vi "sort and index.vi"(2 "Reverse":bool, 3 "Array to Sort":string[](array[string])) -> (0 "Sorted Indices Array":i32[](array[numeric]), 1 "Sorted Array":string[](array[string]))   [LabVIEW 2015]
doc: "This example VI will sort a 1D array and provide an Index Matrix.\n\nFor example:\n\nunsorted array A=[5 4 5 3 1 2]\nsorted array B = [1 2 3 4 5 5]\nIndex Array = [4 5 3 1 0 2]"
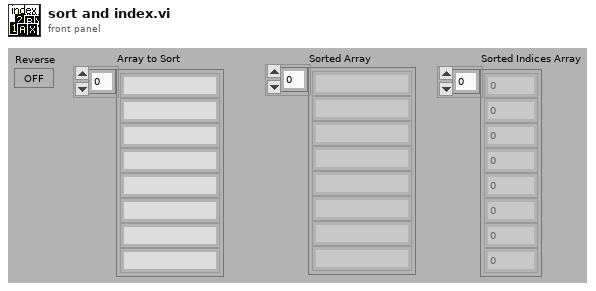
[diagram p1: front panel]
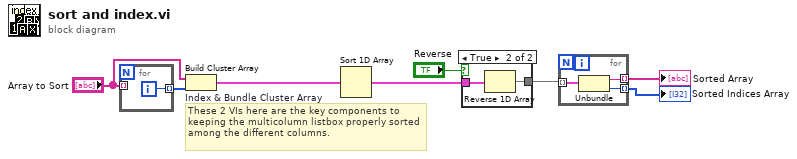
[diagram p0: block diagram]
diagram:
  # "These 2 VIs here are the key components to keeping the multicolumn listbox properly sorted among the different columns."
  n1 = for {
    tunnel: [w9] -> w7 mode=indexing
    tunnel: "Array to Sort" -> [_] mode=indexing
    i -> [w9]
  }
  n2 = Build Cluster Array "Index & Bundle Cluster Array"("Array to Sort", w7) -> (w8:cluster{"String":string, i32}[])
  n3 = Sort 1D Array(array=w8) -> (sorted array=w6:cluster{"String":string, i32}[])
  n4 = case shown="True" "Reverse" {
    tunnel: w6 -> [w10 w12]
    tunnel: [w10 w11] -> w5
    frame False {
    }
    frame True {
      n5 = Reverse 1D Array(array=w12) -> (reversed array=w11:cluster{"String":string, i32}[])
    }
  }
  n6 = for {
    tunnel: w5 -> [w15] mode=indexing
    tunnel: [w14] -> w3 mode=indexing
    tunnel: [w13] -> w2 mode=indexing
    n7 = Unbundle(w15) -> ("String"=w14:string, w13:i32)
  }
  "Sorted Array" <- w3
  "Sorted Indices Array" <- w2
